vi "Create Software Items and Aliases.vi"(8 "error in":errorcluster) -> (0 "error out":errorcluster, 4 "log":string)   [LabVIEW 2024]
uses:
  <vilib>/Plug-In SDKs/Clients/Metadata/Software Item.ctl
  <vilib>/Plug-In SDKs/Clients/Metadata/Extension Value.ctl
  <vilib>/Plug-In SDKs/Clients/Metadata Store V1/Metadata Store Client.lvlibp/API/Metadata Store V1/Create Software Item.vi
  <vilib>/Plug-In SDKs/Clients/Metadata Store V1/Metadata Store Client.lvlibp/API/Metadata Store V1/Create Alias (Metadata - Software Item).vi
  <vilib>/Plug-In SDKs/Clients/Metadata Store V1/Metadata Store Client.lvlibp
  <vilib>/Plug-In SDKs/Clients/Metadata/NI Metadata Types.lvlib
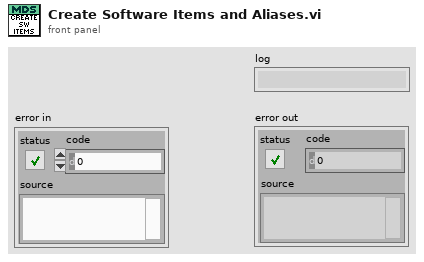
[diagram p1: front panel]
types:
  T1 = typedef "NI Metadata Types.lvlib/Software Item.ctl" = cluster{"product":string, "version":string, "id":string, "link":string, "extension":T2[], "schema id":string}
  T2 = typedef "NI Metadata Types.lvlib/Extension Value.ctl" = cluster{"name":string, "value":string}
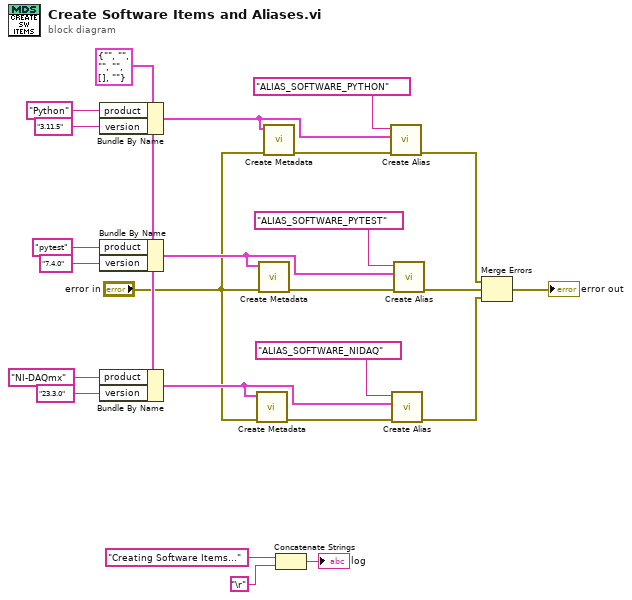
[diagram p0: block diagram]
diagram:
  w6 = T1 {"product"="", "version"="", "id"="", "link"="", "extension"=[], "schema id"=""} ("software item")
  n1 = Bundle By Name(cluster=w6, "product"="Python" ("operator name"), "version"="3.11.5" ("operator name")) -> (w18:T1)
  n2 = Bundle By Name(cluster=w6, "product"="pytest" ("serial number"), "version"="7.4.0" ("model")) -> (w21:T1)
  n3 = Bundle By Name(cluster=w6, "product"="NI-DAQmx" ("serial number"), "version"="23.3.0" ("model")) -> (w7:T1)
  n4 = call-poly <vilib>:"Create Metadata.vi"("error in"="error in", "software item"=w7) -> ("error out"=w9:errorcluster)  [unwired: 8 in, 1 out]
  n5 = call-poly <vilib>:"Create Metadata.vi"("error in"="error in", "software item"=w21) -> ("error out"=w16:errorcluster)  [unwired: 8 in, 1 out]
  n6 = call-poly <vilib>:"Create Metadata.vi"("error in"="error in", "software item"=w18) -> ("error out"=w17:errorcluster)  [unwired: 8 in, 1 out]
  n7 = Concatenate Strings("Creating Software Items..." ("role"), "\r") -> (→"log":string)
  n8 = call-poly <vilib>:"Create Alias.vi"("error in"=w17, "software item"=w18, "alias name"="ALIAS_SOFTWARE_PYTHON") -> ("error out"=w22:errorcluster)  [unwired: 7 in, 1 out]
  n9 = call-poly <vilib>:"Create Alias.vi"("error in"=w9, "software item"=w7, "alias name"="ALIAS_SOFTWARE_NIDAQ") -> ("error out"=w4:errorcluster)  [unwired: 7 in, 1 out]
  n10 = call-poly <vilib>:"Create Alias.vi"("error in"=w16, "software item"=w21, "alias name"="ALIAS_SOFTWARE_PYTEST") -> ("error out"=w23:errorcluster)  [unwired: 7 in, 1 out]
  n11 = Merge Errors(w22, w23, w4) -> (→"error out":errorcluster)
